vi "Create File.vi"(8 "error in (no error)":errorcluster, 10 "File Name Prefix":string) -> (0 "error out":errorcluster, 3 "refnum out":refnum<file>)   [LabVIEW 2015]
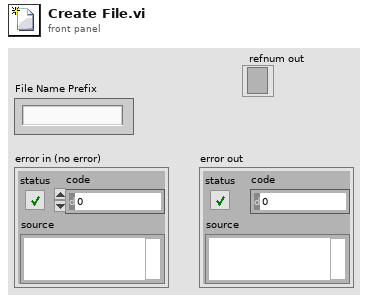
[diagram p1: front panel]
types:
  T1 = enum16{"open", "replace", "create", "open or create", "replace or create", "replace or create with confirmation"}
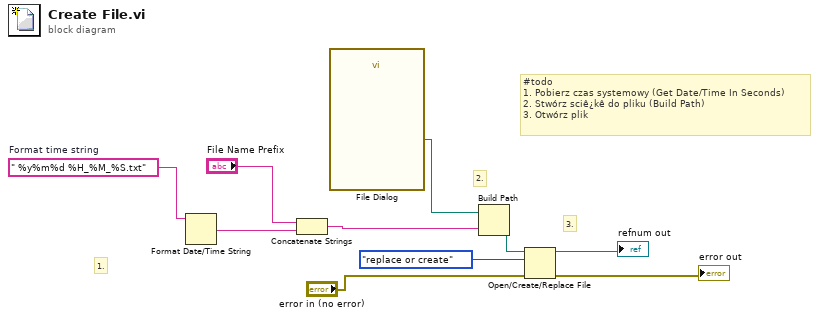
[diagram p0: block diagram]
diagram:
  w9 = " %y%m%d %H_%M_%S.txt"  # Format time string
  # "3."
  # "2."
  # "1."
  # "#todo\n1. Pobierz czas systemowy (Get Date/Time In Seconds)\n2. Stwórz sciê¿kê do pliku (Build Path)\n3. Otwórz plik"
  n1 = Format Date/Time String(time format string (%c)=w9) -> (date/time string=w10:string)  [unwired: 2 in]
  n2 = Concatenate Strings("File Name Prefix", w10) -> (w6:string)
  n3 = call "File Dialog"() -> ("selected path"=w7:path)  [unwired: 12 in, 3 out]
  n4 = Build Path(base path=w7, name or relative path=w6) -> (appended path=w2:path)
  n5 = Open/Create/Replace File(file path (use dialog)=w2, error in="error in (no error)", operation (0:open)=T1."replace or create") -> (refnum out=→"refnum out":refnum<file>, error out=→"error out":errorcluster)  [unwired: 3 in, 1 out]
